vi "lab4_1.vi"() -> ()   [LabVIEW 2021]
panel:
  out "Thermometer 2":dbl(slide) scale=0.0..100.0
  in  "Thermometer":dbl(slide) scale=0.0..100.0
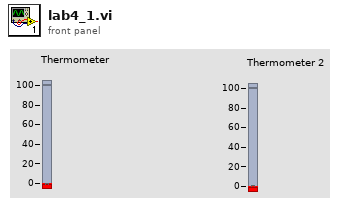
[diagram p1: front panel]
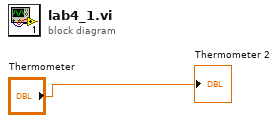
[diagram p0: block diagram]
diagram:
  "Thermometer 2" <- "Thermometer"
